vi "Test TCRS Temperature Ramping Up.vi"(8 "error in (no error)":errorcluster, 11 "Thermal Chamber Response Simlator Test In":refnum<class "Thermal Chamber Response Simlator Test.lvclass">) -> (0 "error out":errorcluster, 3 "Thermal Chamber Response Simlator Test Out":refnum<class "Thermal Chamber Response Simlator Test.lvclass">)   [LabVIEW 2020, in "Thermal Chamber Response Simlator Test.lvclass"]
uses:
  Thermal Chamber Response Simlator Test.lvclass
  C:/Program Files (x86)/National Instruments/LabVIEW 2020/vi.lib/Astemes/LUnit/Test Case.lvclass
  Thermal Chamber Response Simlator/Thermal Chamber Response Simlator.lvclass
  Thermal Chamber Response Simlator/Thermal Chamber Response Simlator.lvclass/Thermal Chamber Response Simlator.ctl
  <vilib>/Astemes/LUnit/Test Case.lvclass/Test Case.ctl
  <vilib>/Astemes/LUnit/LUnit Assertion Result.lvclass/LUnit Assertion Result.ctl
  <vilib>/Astemes/LUnit/LUnit Test Case Result.lvclass/LUnit Test Case Result.ctl
  <vilib>/Astemes/LUnit/LUnit Method Result.lvclass/LUnit Method Result.ctl
  <vilib>/Astemes/LUnit/Palette/Pass If Equal.vi/cbf50e99-f124-4847-863a-8e9794d3dede.vi
  <vilib>/Astemes/LUnit/Palette/Pass.vi
  <vilib>/Astemes/LUnit/Palette/Fail.vi
  <vilib>/Astemes/LUnit/Compare Variants.vi
  <vilib>/Astemes/LUnit/Describe Comparison.vi
  <vilib>/Astemes/LUnit/Set Assertion Type.vi
  <vilib>/Astemes/LUnit/Add test result.vi
  <vilib>/Astemes/LUnit/LUnit Write Passed.vi
  <vilib>/Astemes/LUnit/LUnit Write Message.vi
  <vilib>/Astemes/LUnit/LUnit Write Description.vi
  <vilib>/Astemes/LUnit/Variant to string.vi
  <vilib>/Astemes/LUnit/LUnit Write Assertion Type.vi
  <vilib>/Astemes/LUnit/LUnit Record Assertion Result.vi
  <vilib>/Astemes/LUnit/LUnit Aggregate Assertion Results.vi
  <vilib>/Astemes/LUnit/Assertion Result/LUnit Read Status.vi
  <vilib>/Astemes/LUnit/LUnit Read Message.vi
  <vilib>/Astemes/LUnit/LUnit Read Description.vi
  <vilib>/Astemes/LUnit/Method Result/LUnit Merge Status.vi
  <vilib>/Astemes/LUnit/LUnit Concatenate result strings.vi
  Thermal Chamber Response Simlator/Private/Get Current Time if Not Set.vi
  <vilib>/Utility/Data Type/Get Type Information.vi
  <vilib>/Utility/LVClass/Get LV Class Name.vi
  <vilib>/Astemes/LUnit/LUnit Assertion Result.lvclass
  <vilib>/Astemes/LUnit/Test Case.lvclass
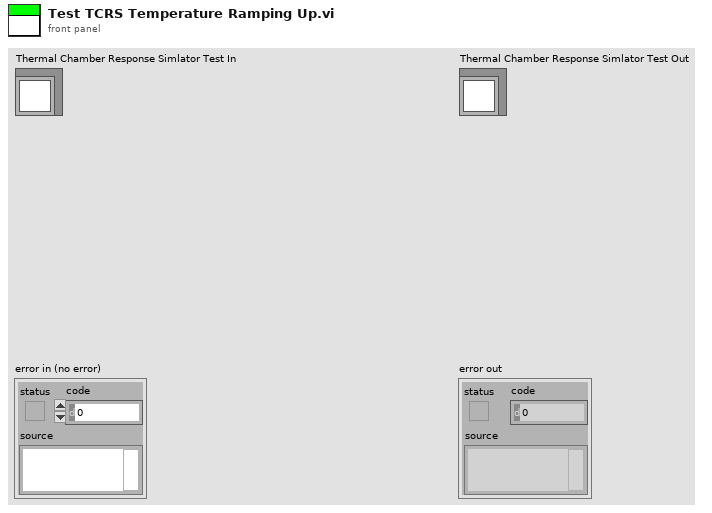
[diagram p1: front panel]
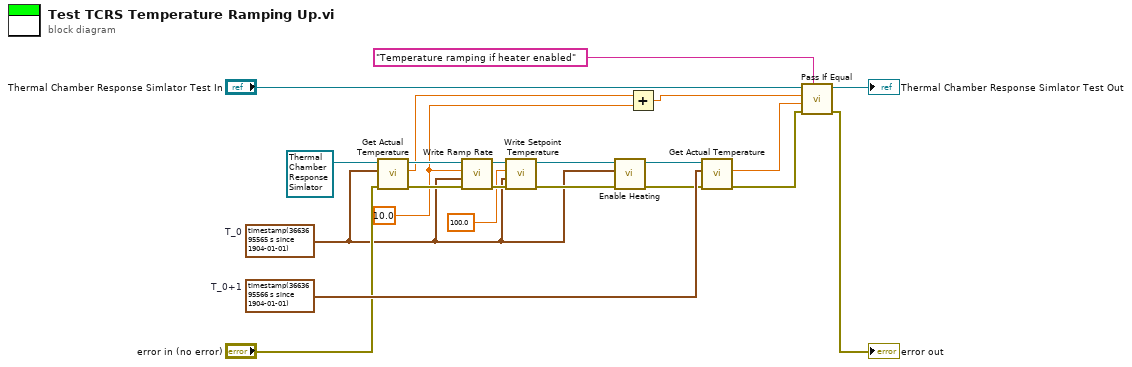
[diagram p0: block diagram]
diagram:
  w17 = timestamp(3663695566 s since 1904-01-01)  # T_0+1
  w6 = 10.0 ("Ramp Rate [degC/s]")
  w1 = timestamp(3663695565 s since 1904-01-01)  # T_0
  n1 = call "Get Actual Temperature.vi"("error in (no error)"="error in (no error)", "Time Stamp"=w1, "Thermal Chamber Response Simlator In"=refnum<class "Thermal Chamber Response Simlator.lvclass"> refnum ("Thermal Chamber Response Simlator.lvclass")) -> ("error out"=w19:errorcluster, "Actual Temperature [degC]"=w13:dbl, "Thermal Chamber Response Simlator Out"=w20:refnum<class "Thermal Chamber Response Simlator.lvclass">)  [unwired: 6 in]
  n2 = call "Write Ramp Rate.vi"("error in (no error)"=w19, "Time Stamp"=w1, "Ramp Rate [degC/s]"=w6, "Thermal Chamber Response Simlator In"=w20) -> ("error out"=w18:errorcluster, "Thermal Chamber Response Simlator Out"=w4:refnum<class "Thermal Chamber Response Simlator.lvclass">)  [unwired: 6 in]
  n3 = call "Write Setpoint Temperature.vi"("error in (no error)"=w18, "Update Time"=w1, "Setpoint Temperature [degC]"=100.0, "Thermal Chamber Response Simlator In"=w4) -> ("error out"=w5:errorcluster, "Thermal Chamber Response Simlator Out"=w3:refnum<class "Thermal Chamber Response Simlator.lvclass">)  [unwired: 6 in]
  n4 = call "Enable Heating.vi"("error in (no error)"=w5, "Start Time"=w1, "Thermal Chamber Response Simlator In"=w3) -> ("error out"=w9:errorcluster, "Thermal Chamber Response Simlator Out"=w8:refnum<class "Thermal Chamber Response Simlator.lvclass">)  [unwired: 7 in]
  n5 = Add(x=w13, y=w6) -> (x+y=w7:dbl)
  n6 = call "Get Actual Temperature.vi"("error in (no error)"=w9, "Time Stamp"=w17, "Thermal Chamber Response Simlator In"=w8) -> ("error out"=w15:errorcluster, "Actual Temperature [degC]"=w14:dbl)  [unwired: 6 in, 1 out]
  n7 = call <vilib>:"Pass If Equal.vi"("Description"="Temperature ramping if heater enabled", "error in (no error)"=w15, "Actual"=w14, "Expected"=w7, "LUnit Test Case In"="Thermal Chamber Response Simlator Test In") -> ("error out"=→"error out":errorcluster, "LUnit Test Case Out"=→"Thermal Chamber Response Simlator Test Out":refnum<class "Thermal Chamber Response Simlator Test.lvclass">)  [unwired: 5 in]
